vi "ZDataVIS_Fix_Filtered_Time.vi"(11 "time array from one itx":dbl[](array[numeric])) -> (3 "fixed itx time array":dbl[](array[numeric]))   [LabVIEW 2016]
uses:
  <vilib>/Analysis/NI_AALPro.lvlib
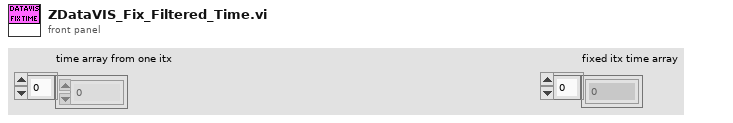
[diagram p1: front panel]
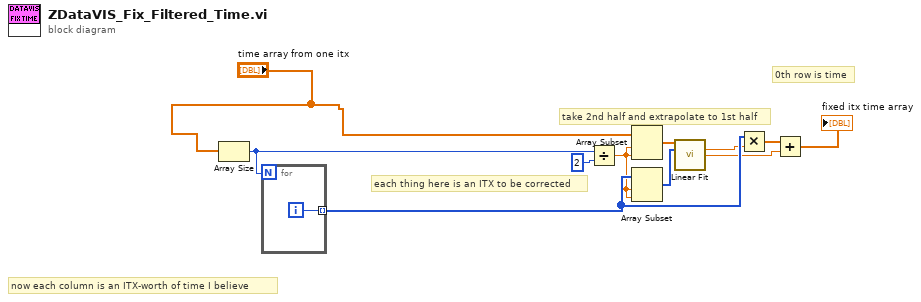
[diagram p0: block diagram]
diagram:
  # "each thing here is an ITX to be corrected"
  # "take 2nd half and extrapolate to 1st half"
  # "now each column is an ITX-worth of time I believe"
  # "0th row is time"
  n1 = Array Size(array="time array from one itx") -> (size(s)=w11:i32)
  n2 = for {
    N: w11 -> [_]
    tunnel: [w12] -> w10 mode=indexing
    i -> [w12]
  }
  n3 = Divide(x=w11, y=2) -> (x/y=w4:dbl)
  n4 = Array Subset(array="time array from one itx", index=w4, length=w4) -> (w5:dbl[])
  n5 = Array Subset(array=w10, index=w4, length=w4) -> (w3:i32[])
  n6 = call <vilib>:"Linear Fit.vi"("Y"=w5, "X"=w3) -> ("slope"=w8:dbl, "intercept"=w6:dbl)  [unwired: 9 in, 3 out]
  n7 = Multiply(x=w10, y=w8) -> (x*y=w7:dbl[])
  n8 = Add(x=w7, y=w6) -> (x+y=→"fixed itx time array":dbl[])
